vi "Load Help File.vi"(8 "error in (no error)":errorcluster, 9 "HTML File to Load":string="MainPage_J1939.html", 10 "Main CHM File":string="J1939.chm", 11 "Browser":refnum<k7>(container)) -> (0 "error out":errorcluster)   [LabVIEW 2021, in "Large Number Operation System Explorer.lvlib"]
doc: "Loads the specified HTML page from the CHM into the browser"
uses:
  Large Number Operation System Explorer.lvlib
  <vilib>/Utility/LVLibp/NI_PackedLibraryUtility.lvlib
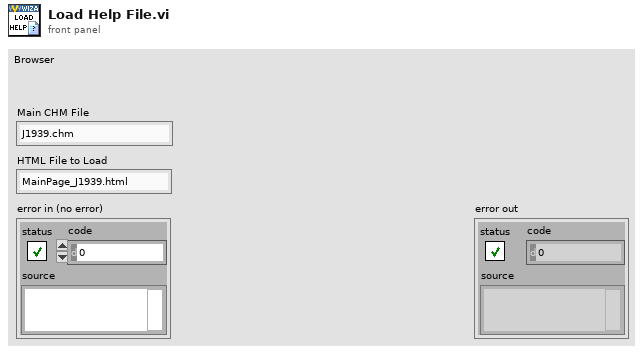
[diagram p1: front panel]
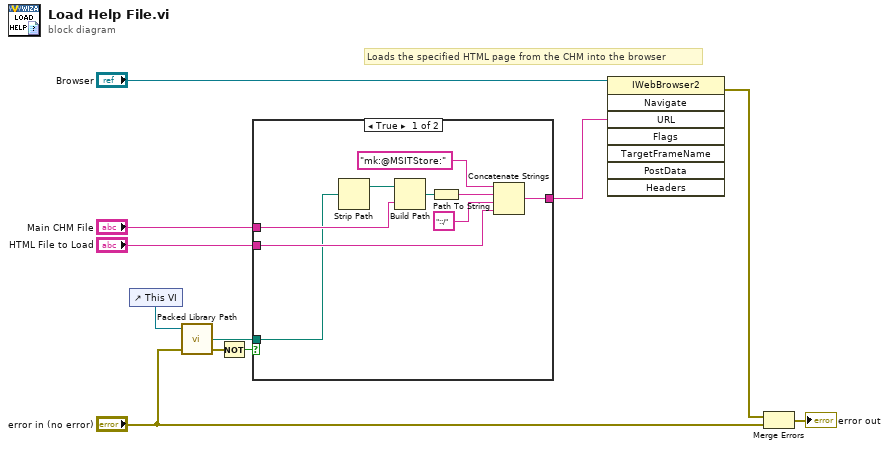
[diagram p0: block diagram]
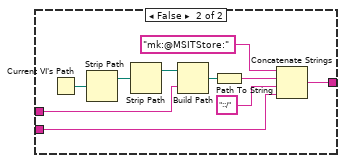
[diagram p2: hidden frame]
diagram:
  # "Loads the specified HTML page from the CHM into the browser"
  n1 = control-ref of="This VI"() -> (w9:refnum<vi>)
  n2 = call <vilib>:"Packed Library Path.vi"("error in (no error)"="error in (no error)", "vi reference"=w9) -> ("error out"=w6:errorcluster, "packed library path"=w8:path)  [unwired: 1 in, 1 out]
  n3 = Not(x=w6) -> (.not. x?=w7:bool)
  n4 = case shown="True" w7 {
    tunnel: "Main CHM File" -> [w16 w24]
    tunnel: [w15 w22] -> w1
    tunnel: "HTML File to Load" -> [w14 w21]
    tunnel: w8 -> [w13 _]
    frame True {
      n5 = Strip Path(path=w13) -> (stripped path=w12:path)  [unwired: 1 out]
      n6 = Build Path(base path=w12, name or relative path=w16) -> (appended path=w17:path)
      n7 = Path To String(path=w17) -> (string=w18:string)
      n8 = Concatenate Strings("mk:@MSITStore:" ("string"), w18, "::/" ("name or relative path"), w14) -> (w15:string)
    }
    frame False {
      n9 = Current VI's Path() -> (path=w29:path)
      n10 = Strip Path(path=w29) -> (stripped path=w28:path)  [unwired: 1 out]
      n11 = Strip Path(path=w28) -> (stripped path=w23:path)  [unwired: 1 out]
      n12 = Build Path(base path=w23, name or relative path=w24) -> (appended path=w25:path)
      n13 = Path To String(path=w25) -> (string=w26:string)
      n14 = Concatenate Strings("mk:@MSITStore:" ("string"), w26, "::/" ("name or relative path"), w21) -> (w22:string)
    }
  }
  n15 = invoke class="IWebBrowser2" method="Navigate"(reference="Browser", "URL"=w1) -> (error out=w3:errorcluster)  [unwired: 6 in, 7 out]
  n16 = Merge Errors(w3, "error in (no error)") -> (→"error out":errorcluster)
